vi "_Monitor.vi"() -> ()   [LabVIEW 2017]
uses:
  Multi-Instance/_DEF-DBOper.ctl
  TagDB(DEV).lvlib
panel:
  out "Count":i32
  in  "Menual Refresh":bool
  in  "Page":enum16{"Common", "Table"}(ring)
  in  "Timeout(ms)":u32=500 min=100 max=60000 step=1
  in  "Auto Refresh?":bool
  in  "DB List":i32(listbox)
  in  "Refresh DB List":bool
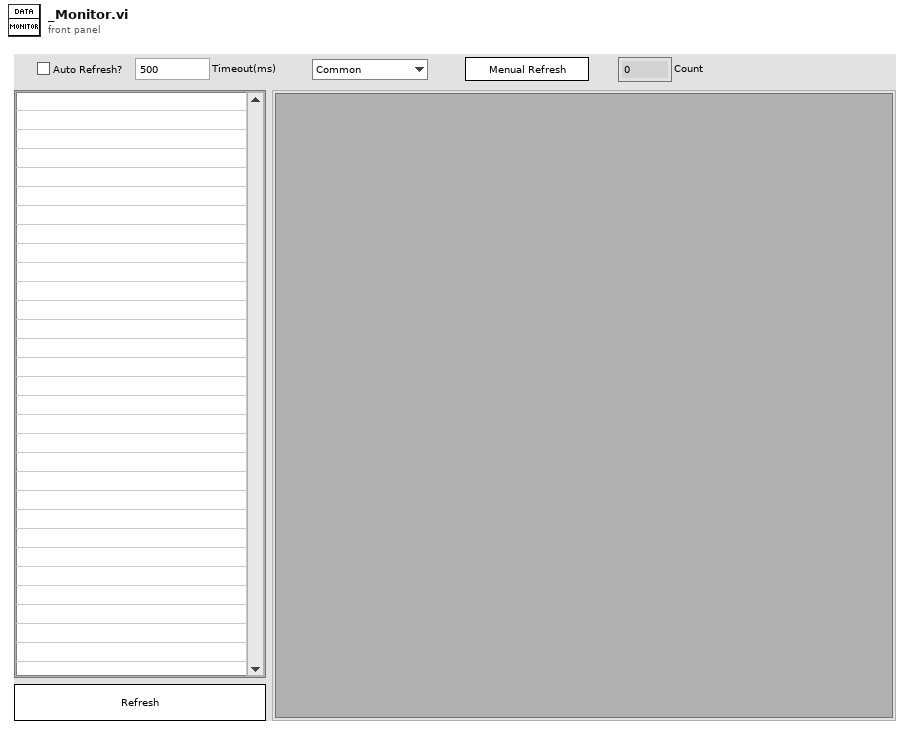
[diagram p1: front panel]
types:
  T1 = cluster{"Sub Panel":refnum<vi>, "DB List":refnum<vi>, "Probe":refnum<vi>, "Tab Probe":refnum<vi>}
  T2 = enum32{"Invalid", "Standard", "Closed", "Hidden", "Minimized", "Maximized"}
  T3 = typedef "TagDB(DEV).lvlib/_DEF-DBOper.ctl" = enum16{"create", "destroy", "cleanUp", "list", "get info"}
  T4 = cluster{"DB List":string[], "Page":enum16{"Common", "Table"}}
  T5 = typedef "TagDB(DEV).lvlib/TagContainer.ctl" = refnum<k1>
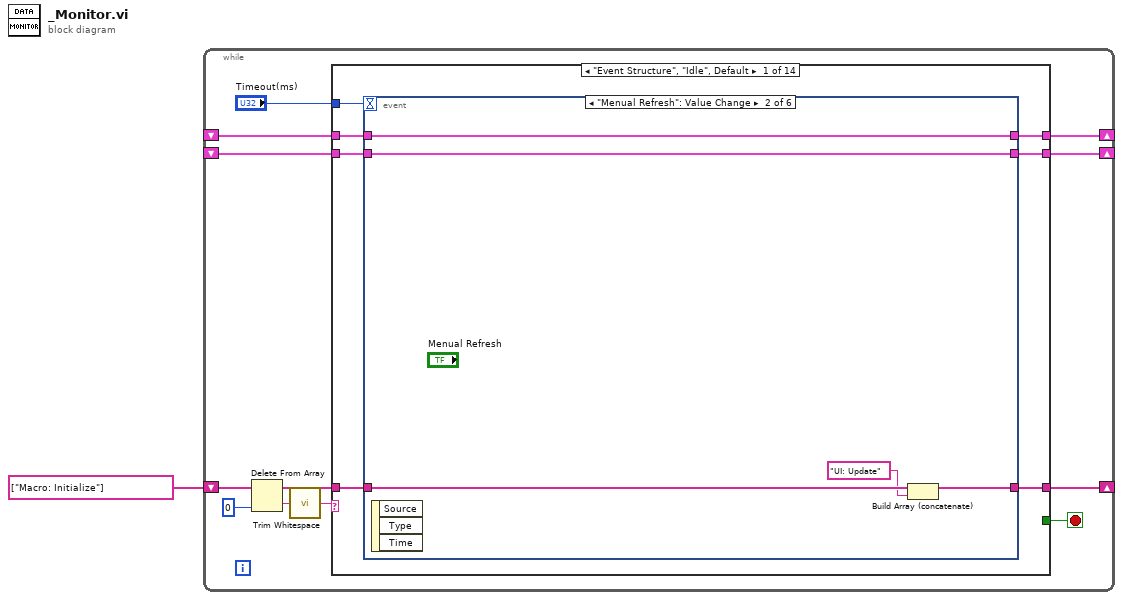
[diagram p0: block diagram]
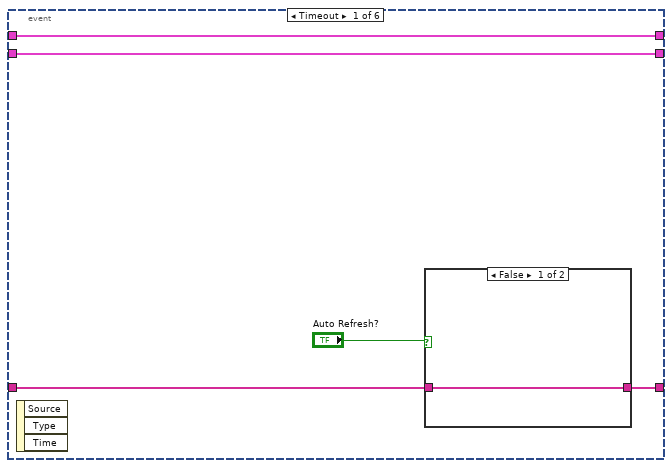
[diagram p2: hidden frame]
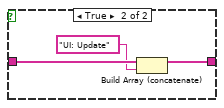
[diagram p3: hidden frame]
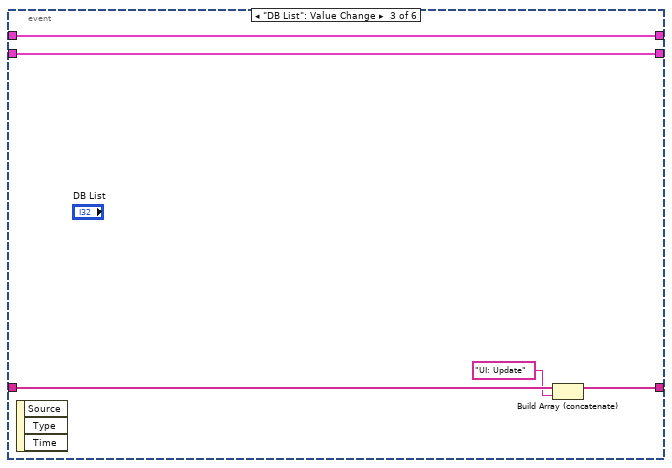
[diagram p4: hidden frame]
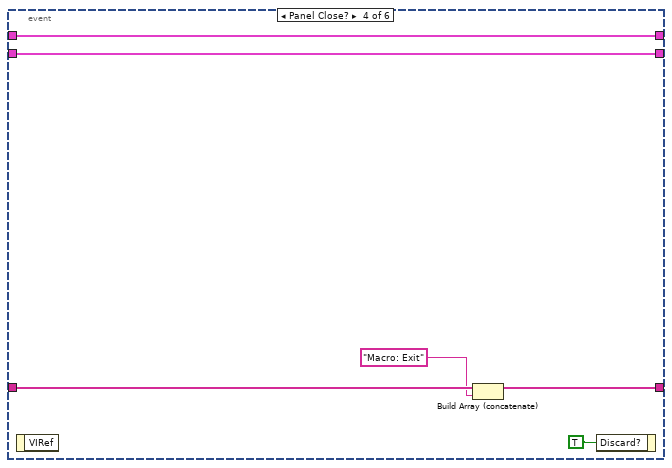
[diagram p5: hidden frame]
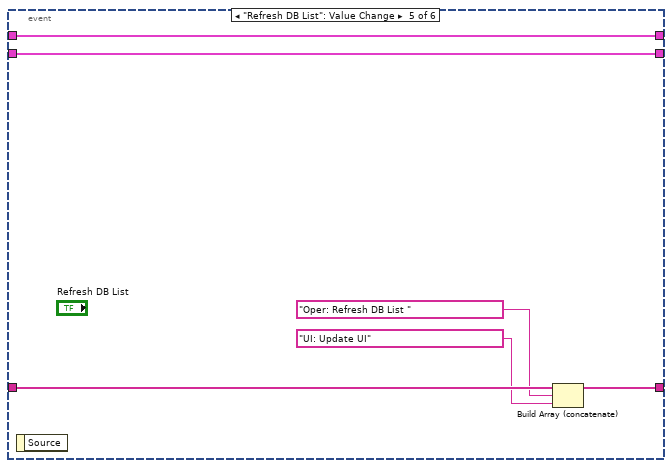
[diagram p6: hidden frame]
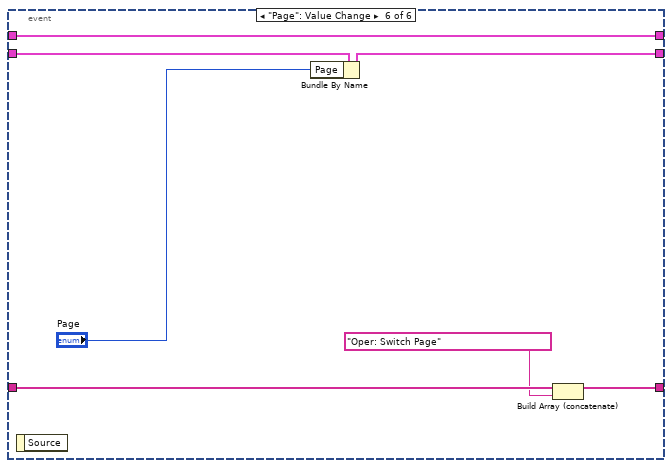
[diagram p7: hidden frame]
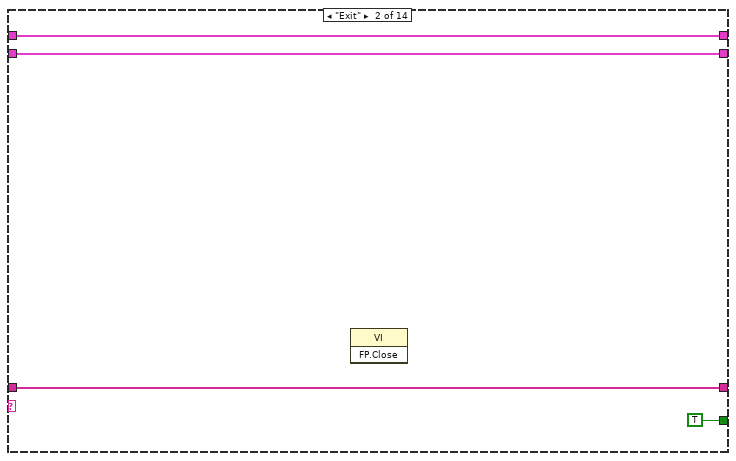
[diagram p8: hidden frame]
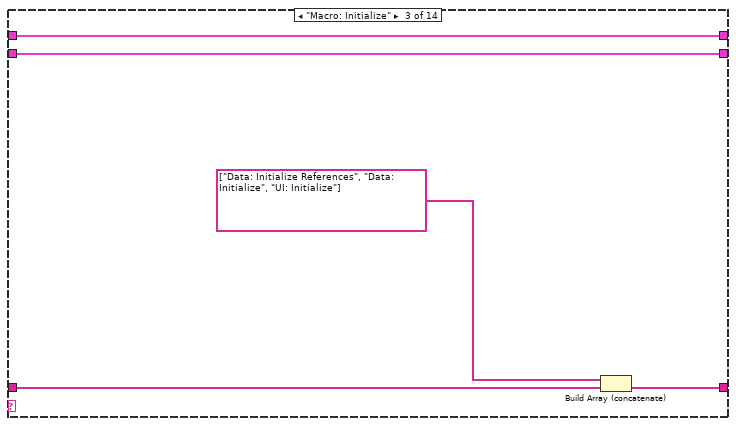
[diagram p9: hidden frame]
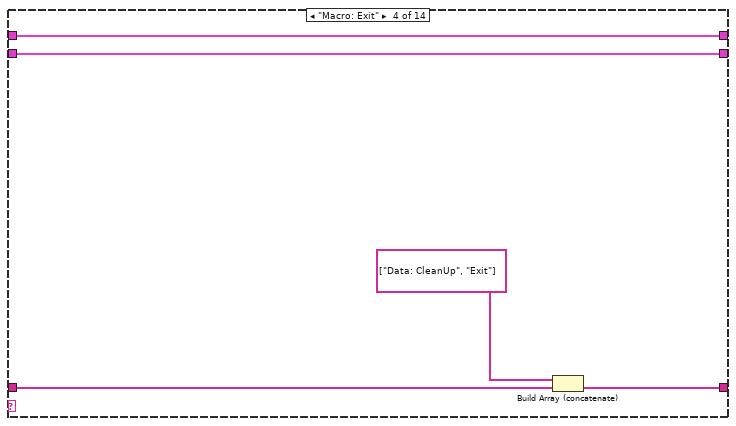
[diagram p10: hidden frame]
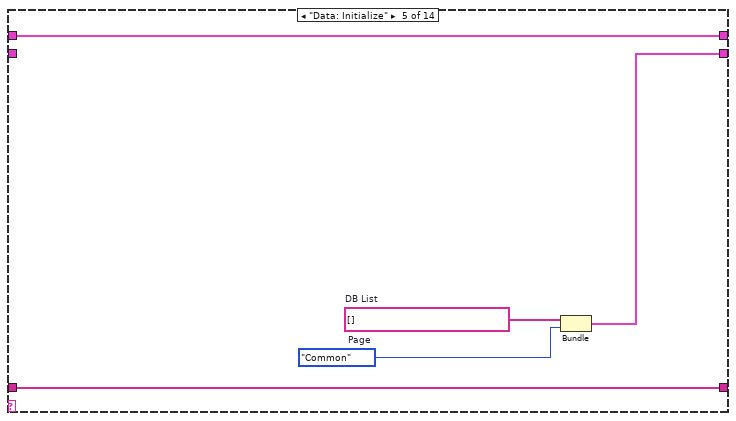
[diagram p11: hidden frame]
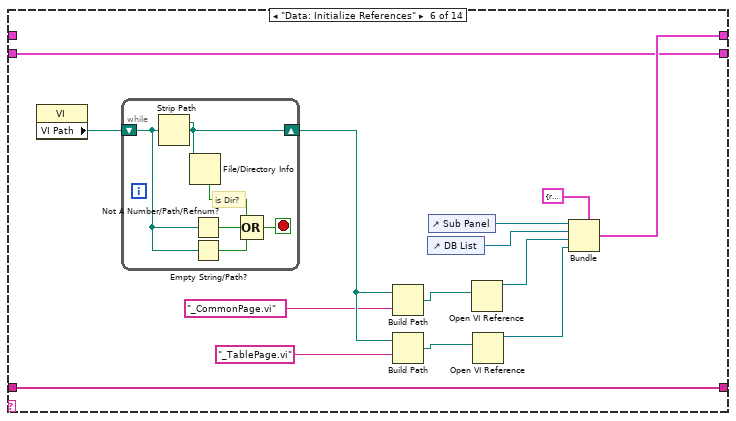
[diagram p12: hidden frame]
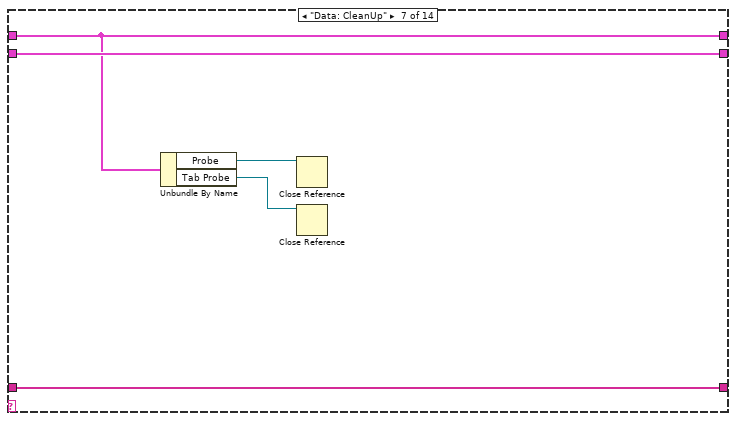
[diagram p13: hidden frame]
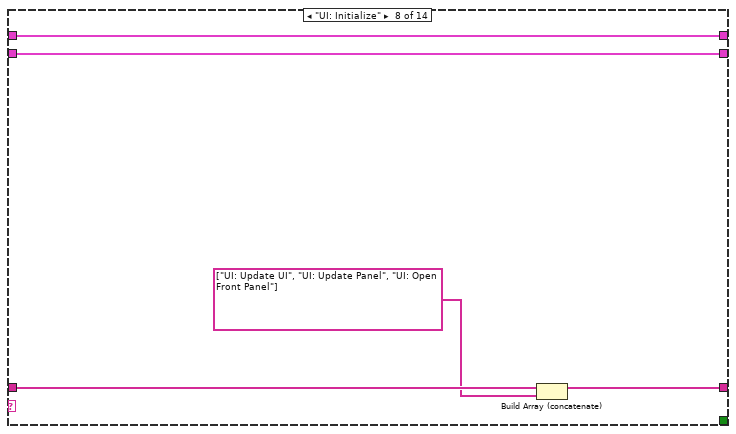
[diagram p14: hidden frame]
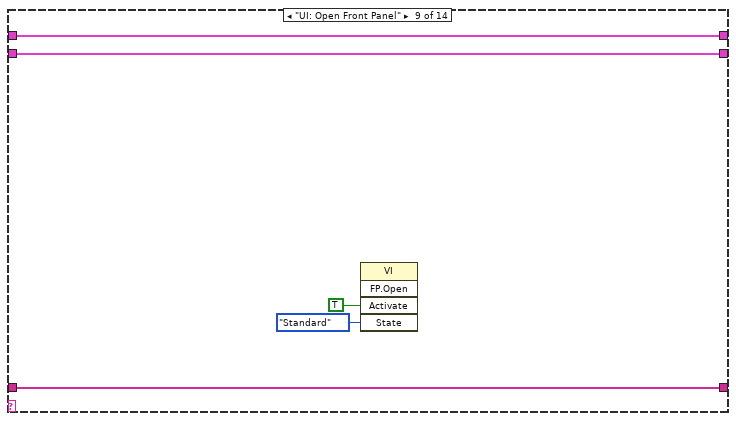
[diagram p15: hidden frame]
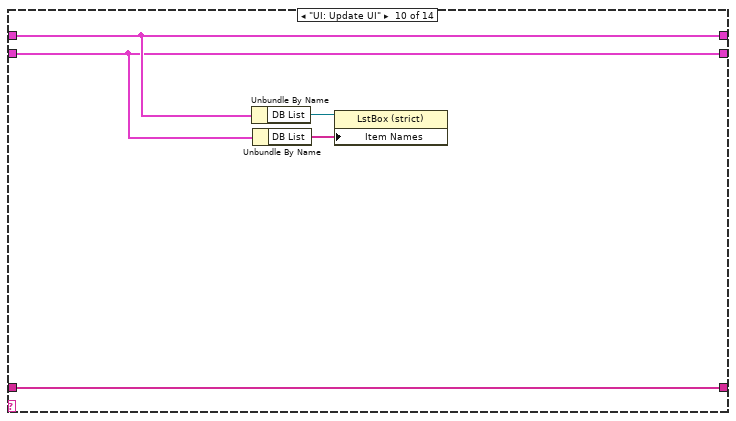
[diagram p16: hidden frame]
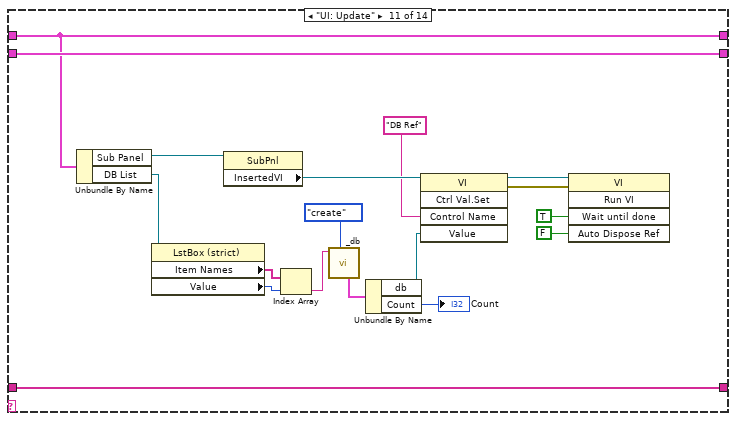
[diagram p17: hidden frame]
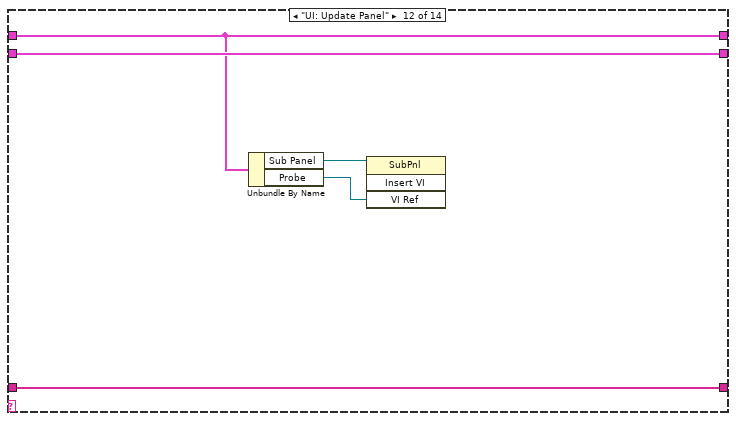
[diagram p18: hidden frame]
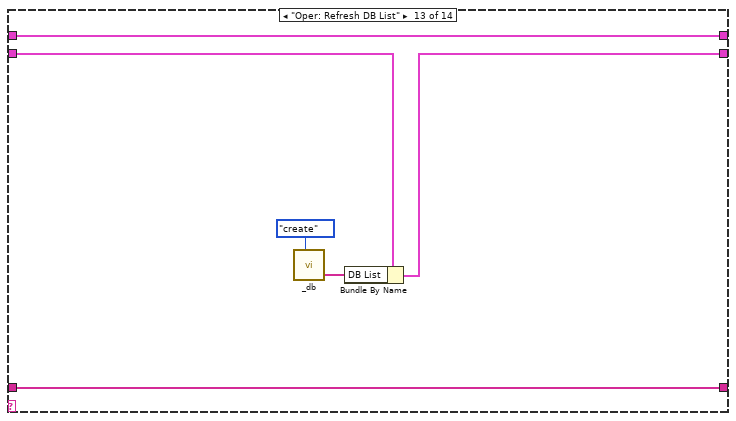
[diagram p19: hidden frame]
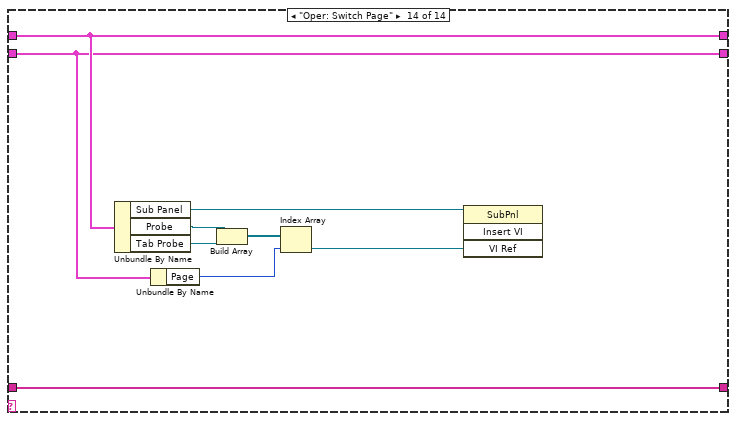
[diagram p20: hidden frame]
diagram:
  n1 = while {
    shift-right: [w8] -> _
    shift-left: string[] ["Macro: Initialize"] -> [w12]
    shift-right: [w7] -> _
    shift-left: _ -> [w6]
    shift-right: [w3] -> _
    shift-left: _ -> [w5]
    stop <- w13 stop-if-true
    n2 = Delete From Array(array=w12, index=0) -> (deleted portion=w11:string, array with subset deleted=w9:string[])  [unwired: 1 in]
    n3 = call <vilib>:"Trim Whitespace.vi"("string"=w11) -> ("trimmed string"=w4:string)  [unwired: 1 in]
    n4 = case shown="\"Event Structure\", \"Idle\", Default" w4 {
      tunnel: [_ TRUE _ _ _ _ _ _ _ _ _ _ _ _] -> w13
      tunnel: w9 -> [w20 w62 w67 w72 w77 w91 w102 w107 w112 w117 w135 w140 w146 w155]
      tunnel: [w19 w62 w64 w69 w77 w91 w102 w104 w112 w117 w135 w140 w146 w155] -> w8
      tunnel: [w16 w61 w66 w71 w75 w83 w101 w106 w111 w114 w134 w139 w144 w150] -> w7
      tunnel: w6 -> [w15 w61 w66 w71 _ w83 w101 w106 w111 w114 w134 w139 w145 w150]
      tunnel: w5 -> [w17 w60 w65 w70 w73 _ w100 w105 w110 w116 w133 w138 w142 w154]
      tunnel: [w18 w60 w65 w70 w73 w88 w100 w105 w110 w116 w133 w138 w142 w154] -> w3
      tunnel: "Timeout(ms)" -> [w14 _ _ _ _ _ _ _ _ _ _ _ _ _]
      frame "Event Structure", "Idle", Default {
        n5 = event shown="[1] \"Menual Refresh\": Value Change" {
          selector: _ -> [_ _ _ _ _ _]
          dyn-events: _ -> [_ _ _ _ _ _]
          timeout: w14 -> [_ _ _ _ _ _]
          tunnel: w20 -> [w25 w34 w39 w44 w51 w58]
          tunnel: [w22 w31 w36 w43 w50 w57] -> w19
          tunnel: [w24 w33 w38 w41 w47 w55] -> w18
          tunnel: w17 -> [w24 w33 w38 w41 w47 w55]
          tunnel: [w23 w32 w37 w40 w46 w53] -> w16
          tunnel: w15 -> [w23 w32 w37 w40 w46 w54]
          event Timeout {
            n6 = event-data() -> ()  [unwired: 1 in, 3 out]
            n7 = case shown="False" "Auto Refresh?" {
              tunnel: w25 -> [w26 w29]
              tunnel: [w26 w28] -> w22
              frame False {
              }
              frame True {
                n8 = Build Array (concatenate)(w29, "UI: Update") -> (w28:string[])
              }
            }
          }
          event "Menual Refresh": Value Change {
            n9 = event-data() -> ()  [unwired: 1 in, 3 out]
            n10 = Build Array (concatenate)(w34, "UI: Update") -> (w31:string[])
          }
          event "DB List": Value Change {
            n11 = event-data() -> ()  [unwired: 1 in, 3 out]
            n12 = Build Array (concatenate)(w39, "UI: Update") -> (w36:string[])
          }
          event Panel Close? {
            n13 = event-data() -> ()  [unwired: 1 in, 1 out]
            n14 = Build Array (concatenate)(w44, "Macro: Exit") -> (w43:string[])
            n15 = event-data("Discard?"=TRUE) -> ()  [unwired: 1 in, 1 out]
          }
          event "Refresh DB List": Value Change {
            n16 = event-data() -> ()  [unwired: 1 in, 1 out]
            n17 = Build Array (concatenate)(w51, "Oper: Refresh DB List ", "UI: Update UI") -> (w50:string[])
          }
          event "Page": Value Change {
            n18 = event-data() -> ()  [unwired: 1 in, 1 out]
            n19 = Bundle By Name(cluster=w54, "Page"="Page") -> (w53:T4)
            n20 = Build Array (concatenate)(w58, "Oper: Switch Page") -> (w57:string[])
          }
        }
      }
      frame "Exit" {
        n21 = invoke class="VI" method="FP.Close"() -> ()  [unwired: 3 in, 3 out]
      }
      frame "Macro: Initialize" {
        n22 = Build Array (concatenate)(string[] ["Data: Initialize References", "Data: Initialize", "UI: Initialize"] ("array"), w67) -> (w64:string[])
      }
      frame "Macro: Exit" {
        n23 = Build Array (concatenate)(string[] ["Data: CleanUp", "Exit"] ("array"), w72) -> (w69:string[])
      }
      frame "Data: Initialize" {
        w74 = enum16{"Common", "Table"}."Common"  # Page
        w76 = string[] []  # DB List
        n24 = Bundle("DB List"=w76, "Page"=w74) -> (w75:T4)  [unwired: 1 in]
      }
      frame "Data: Initialize References" {
        n25 = property class="VI"() -> ("VI Path"=w84:path)  [unwired: 2 in, 2 out]
        n26 = while {
          shift-right: [w92] -> w80
          shift-left: w84 -> [w94]
          stop <- w96 stop-if-true
          # "is Dir?"
          n27 = Strip Path(path=w94) -> (stripped path=w92:path)  [unwired: 1 out]
          n28 = File/Directory Info(path=w92) -> (directory=w97:bool)  [unwired: 1 in, 6 out]
          n29 = Not A Number/Path/Refnum?(number/path/refnum=w94) -> (NaN/Path/Refnum?=w95:bool)
          n30 = Empty String/Path?(string/path=w94) -> (empty?=w93:bool)
          n31 = Compound Arithmetic op=OR(w97, w95, w93) -> (w96:bool)
        }
        n32 = Build Path(base path=w80, name or relative path="_CommonPage.vi") -> (appended path=w82:path)
        n33 = Build Path(base path=w80, name or relative path="_TablePage.vi") -> (appended path=w81:path)
        n34 = control-ref of="DB List"() -> (w89:refnum<vi>)
        n35 = control-ref of="Sub Panel"() -> (w90:refnum<vi>)
        n36 = Open VI Reference(vi path=w82) -> (vi reference=w85:refnum<vi>)  [unwired: 5 in, 1 out]
        n37 = Open VI Reference(vi path=w81) -> (vi reference=w86:refnum<vi>)  [unwired: 5 in, 1 out]
        n38 = Bundle(cluster=T1 {"Sub Panel"=refnum, "DB List"=refnum, "Probe"=refnum, "Tab Probe"=refnum}, "Sub Panel"=w90, "DB List"=w89, "Probe"=w85, "Tab Probe"=w86) -> (w88:T1)
      }
      frame "Data: CleanUp" {
        n39 = Unbundle By Name(w100) -> ("Probe"=w99:refnum<vi>, "Tab Probe"=w98:refnum<vi>)
        n40 = Close Reference(reference=w99) -> ()  [unwired: 1 in, 1 out]
        n41 = Close Reference(reference=w98) -> ()  [unwired: 1 in, 1 out]
      }
      frame "UI: Initialize" {
        n42 = Build Array (concatenate)(w107, string[] ["UI: Update UI", "UI: Update Panel", "UI: Open Front Panel"] ("array")) -> (w104:string[])
      }
      frame "UI: Open Front Panel" {
        n43 = invoke class="VI" method="FP.Open"("Activate"=TRUE ("Activate?"), "State"=T2."Standard") -> ()  [unwired: 3 in, 5 out]
      }
      frame "UI: Update UI" {
        n44 = Unbundle By Name(w116) -> ("DB List"=w115:refnum<vi>)
        n45 = Unbundle By Name(w114) -> ("DB List"=w113:string[])
        n46 = property class="LstBox (strict)"(reference=w115, "Item Names"=w113) -> ()  [unwired: 1 in, 2 out]
      }
      frame "UI: Update" {
        n47 = Unbundle By Name(w133) -> ("Sub Panel"=w132:refnum<vi>, "DB List"=w130:refnum<vi>)
        n48 = property class="LstBox (strict)"(reference=w130) -> ("Item Names"=w129:string[], "Value"=w128:i32)  [unwired: 1 in, 2 out]
        n49 = property class="SubPnl"(reference=w132) -> ("InsertedVI"=w131:refnum<vi>)  [unwired: 1 in, 2 out]
        n50 = Index Array(array=w129, index=w128) -> (element=w127:string)
        n51 = call "_db.vi"("command"=_DEF-DBOper."create", "name"=w127) -> ("info"=w121:cluster{"db":T5, "Count":i32})  [unwired: 5 in, 4 out]
        n52 = Unbundle By Name(w121) -> ("db"=w120:T5, "Count"=→"Count":i32)
        n53 = invoke class="VI" method="Ctrl Val.Set"(reference=w131, "Control Name"="DB Ref", "Value"=w120) -> (reference out=w125:refnum<vi>, error out=w124:errorcluster)  [unwired: 2 in, 3 out]
        n54 = invoke class="VI" method="Run VI"(reference=w125, error in=w124, "Wait until done"=TRUE ("Wait Until Done"), "Auto Dispose Ref"=FALSE ("Auto Dispose Reference")) -> ()  [unwired: 1 in, 5 out]
      }
      frame "UI: Update Panel" {
        n55 = Unbundle By Name(w138) -> ("Sub Panel"=w137:refnum<vi>, "Probe"=w136:refnum<vi>)
        n56 = invoke on="Invoke Node" class="SubPnl" method="Insert VI"(reference=w137, "VI Ref"=w136) -> ()  [unwired: 2 in, 4 out]
      }
      frame "Oper: Refresh DB List" {
        n57 = call "_db.vi"("command"=_DEF-DBOper."create") -> ("db list"=w143:string[])  [unwired: 6 in, 4 out]
        n58 = Bundle By Name(cluster=w145, "DB List"=w143) -> (w144:T4)
      }
      frame "Oper: Switch Page" {
        n59 = Unbundle By Name(w154) -> ("Sub Panel"=w148:refnum<vi>, "Probe"=w153:refnum<vi>, "Tab Probe"=w152:refnum<vi>)
        n60 = Unbundle By Name(w150) -> ("Page"=w149:enum16{"Common", "Table"})
        n61 = Build Array(w153, w152) -> (w151:refnum<vi>[])
        n62 = Index Array(array=w151, index=w149) -> (element=w147:refnum<vi>)
        n63 = invoke class="SubPnl" method="Insert VI"(reference=w148, "VI Ref"=w147) -> ()  [unwired: 2 in, 4 out]
      }
    }
  }
